vi "XML_fast.vi"(6 "Channel Cluster":T3={"det_type"=[], "voltage"=[], "Serial numbers"=[], "Sources"=[], "Trigger level"=[4000, 4000, 4000, 4000, 4000, 4000, 4000, 4000], "Channel On/Off"=[], "Number of Channels"=8}, 7 "DAQ Info Cluster":T1={"Data Chunks per File"=1000, "Samples per Waveform"=95, "Pretrigger Samples"=15, "circular buffer length (samples)"=1000, "Waveforms per Data Chunk"=5000} {"Waveforms per Data Chunk" format="%.2p"}, 8 "Testpulse Cluster":T2={"Master Pulser On/Off"=FALSE, "Testpulse Turnaround Time (samples)"=14, "Pulse Separation (samples)"=0, "Pulse duration (samples)"=0}, 9 "IP Address of NIST Time Server":string(combo), 10 "NIST Time":u64, 11 "General Cluster":cluster{"Location":i16} {"Location" items=["Purdue", "NIKHEF", "Zurich", "???"]}) -> (2 "XML String":string)   [LabVIEW 2012]
panel:
  # "Waveform/Data Chunk information"
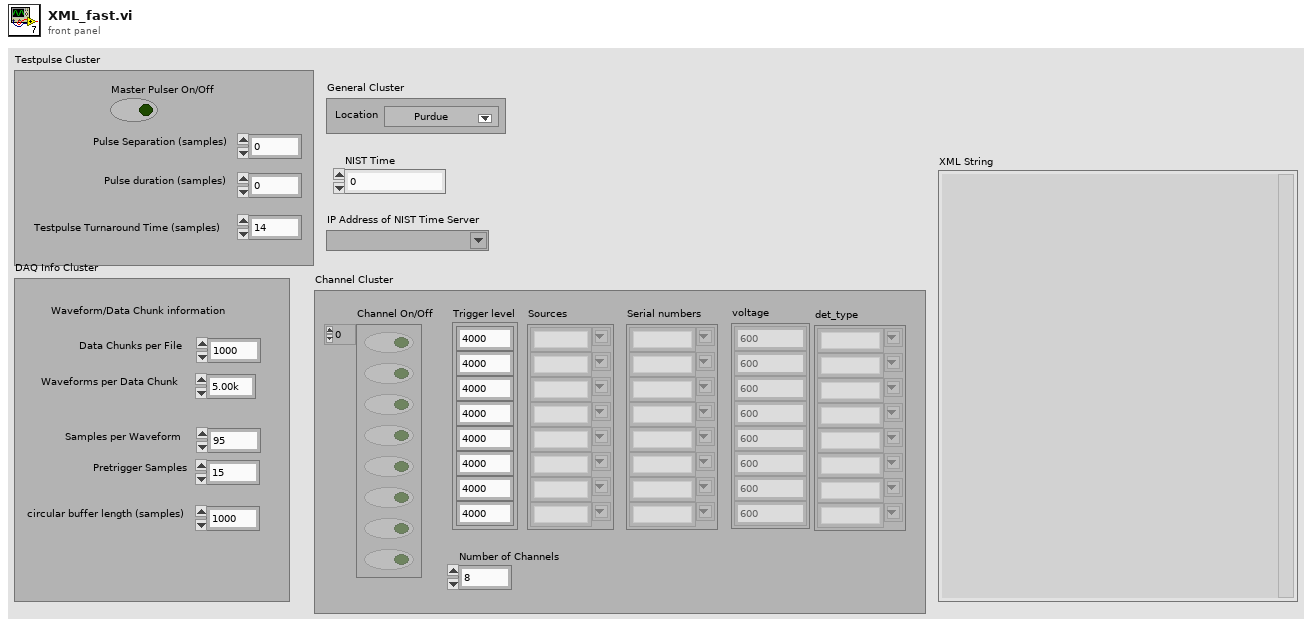
[diagram p1: front panel]
types:
  T1 = cluster{"Data Chunks per File":u32, "Samples per Waveform":u32, "Pretrigger Samples":u32, "circular buffer length (samples)":u32, "Waveforms per Data Chunk":u32}
  T2 = cluster{"Master Pulser On/Off":bool, "Testpulse Turnaround Time (samples)":u32, "Pulse Separation (samples)":u32, "Pulse duration (samples)":u32}
  T3 = cluster{"det_type":string[], "voltage":string[], "Serial numbers":string[], "Sources":string[], "Trigger level":i16[], "Channel On/Off":bool[], "Number of Channels":u8}
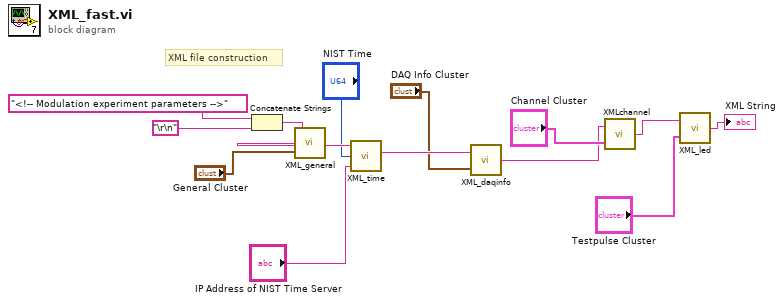
[diagram p0: block diagram]
diagram:
  # "XML file construction"
  n1 = Concatenate Strings("<!-- Modulation experiment parameters -->", "\r\n") -> (w7:string)
  n2 = call "XML_general.vi"("General Cluster"="General Cluster", "Input String"=w7) -> ("Output String"=w6:string)
  n3 = call "XML_time.vi"("IP Address of NIST Time Server"="IP Address of NIST Time Server", "NIST Time"="NIST Time", "Input String"=w6) -> ("Output String"=w5:string)
  n4 = call "XML_daqinfo.vi"("DAQ Info Cluster"="DAQ Info Cluster", "Input String"=w5) -> ("Output String"=w4:string)
  n5 = call "XMLchannel.vi"("Channel Cluster"="Channel Cluster", "Previous XML string"=w4) -> ("Output String"=w10:string)
  n6 = call "XML_led.vi"("Testpulse Cluster"="Testpulse Cluster", "Input String"=w10) -> ("Output String"=→"XML String":string)
